vi "Blinking Boolean.vi"(6 "Error In":errorcluster, 8 "Color 2 (Background, Foreground)":cluster{u32, u32}[](array[cluster])=[{32639, 4587330}], 9 "Color 1 (Background, Foreground)":cluster{u32, u32}[](array[cluster])=[{32639, 4587330}], 10 "Shift in":bool=TRUE, 11 "Bool Refnum":refnum<vi>) -> (0 "Error Out":errorcluster, 2 "Shift out":bool, 3 "reference out":refnum<vi>)   [LabVIEW 2014, in "Display Panel.lvlib"]
uses:
  Generic Instrument/Display Panel/Display Panel.lvlib
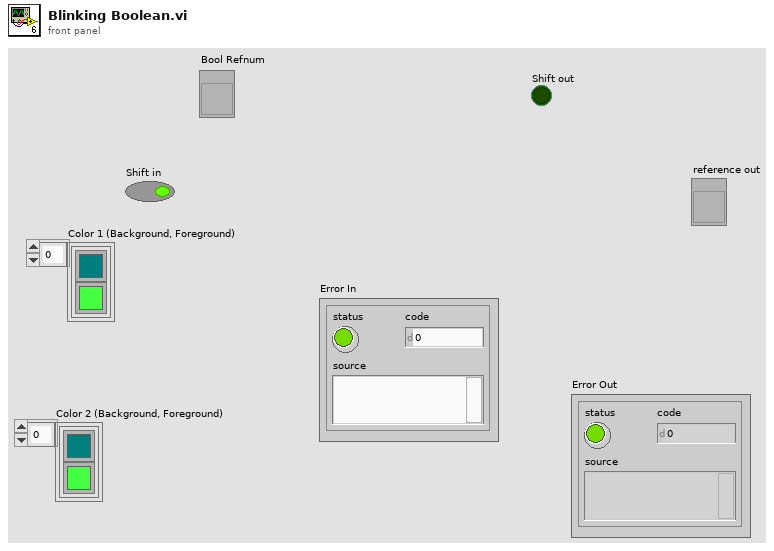
[diagram p1: front panel]
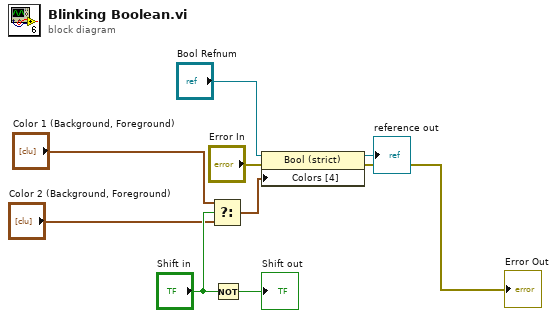
[diagram p0: block diagram]
diagram:
  n1 = Select(t="Color 1 (Background, Foreground)", s="Shift in", f="Color 2 (Background, Foreground)") -> (s? t:f=w4:cluster{u32, u32}[])
  n2 = Not(x="Shift in") -> (.not. x?=→"Shift out":bool)
  n3 = property class="Bool (strict)"(reference="Bool Refnum", error in="Error In", "Colors [4]"=w4) -> (reference out=→"reference out":refnum<vi>, error out=→"Error Out":errorcluster)
